vi "LJM startup config check.vi"(8 "Good Config?":bool, 11 "Config Error In":errorcluster) -> (2 "Force Defaults":bool)   [LabVIEW 2025]
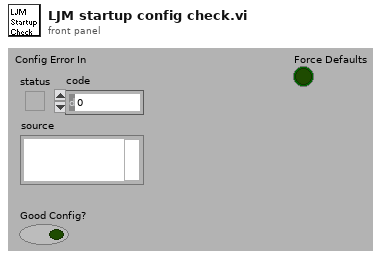
[diagram p1: front panel]
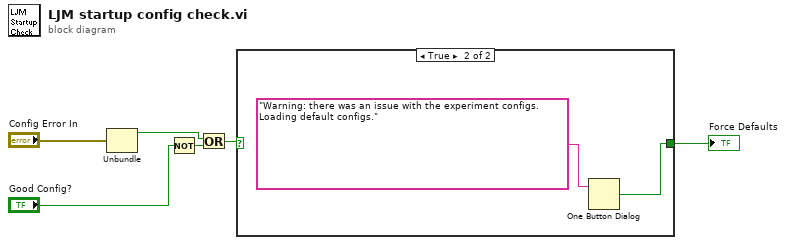
[diagram p0: block diagram]
diagram:
  n1 = Unbundle("Config Error In") -> ("status"=w3:bool)  [unwired: 2 out]
  n2 = Not(x="Good Config?") -> (.not. x?=w5:bool)
  n3 = Or(x=w3, y=w5) -> (x .or. y?=w2:bool)
  n4 = case shown="True" w2 {
    selector: w2 -> [w7 _]
    tunnel: [w7 w9] -> w1
    frame False {
    }
    frame True {
      n5 = One Button Dialog(message="Warning: there was an issue with the experiment configs. Loading default configs.") -> (true=w9:bool)  [unwired: 1 in]
    }
  }
  "Force Defaults" <- w1
